vi "Dkm To Sxx Bare.vi"(8 "error in (no error)":errorcluster, 10 "units":i32, 11 "dKilo":dbl) -> (0 "error out":errorcluster, 3 "function return":string)   [LabVIEW 2023, in "POSCONV.lvlib"]
doc: "char *DkmToSxxBare(double dKilo, int units);"
uses:
  POSCONV.lvlib
  C:/Users/J Gordon/Documents/Rail Tech/TV-HR/02 - Code/Modules/POSCONV/POSCONV.dll
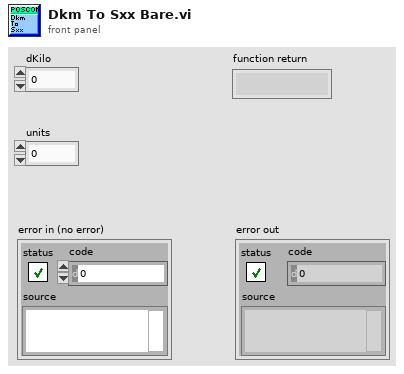
[diagram p1: front panel]
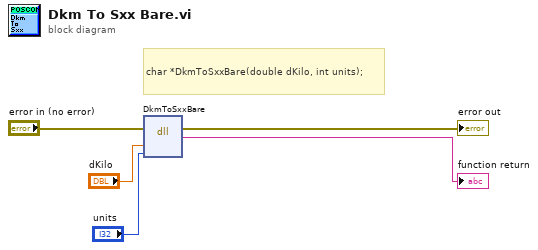
[diagram p0: block diagram]
diagram:
  # "char *DkmToSxxBare(double dKilo, int units);"
  n1 = dll-call lib="C:/Users/J Gordon/Documents/Rail Tech/TV-HR/02 - Code/Modules/POSCONV/POSCONV.*" fn="DkmToSxxBare"(error in="error in (no error)", "dKilo"="dKilo", "units"="units") -> (error out=→"error out":errorcluster, →"function return":string)  [unwired: 4 in, 1 out]
